vi "5GNR_DPD_AMPM_EVM_ACP_DL.vi"() -> ()   [LabVIEW 2016]
doc: "This example illustrates how to use the RFmx SpecAn and LTE personalities together with the RFSG drivers to perform ACP and EVM measurements with or without digital predistortion (DPD) of the waveform input to the DUT. \n\nDPD is a technique to optimize the operating point of power amplifiers and other non-linear RFIC devices. Power amplifiers are much more efficient if they operate near compression. However, compressing signal amplitudes can significantly deteriorate the amplified signal's quality both, in-band (e.g., EVM increases due to non-linear distortion of the signal's I/Q constellation) and out-of-band (e.g., ACP or SEM test fails due to spectral regrowth). With DPD, the original waveform is first pre-distorted in a way that matches the non-linear effects of the RFIC device before being fed through the device. The resulting output is a much cleaner amplified and/or filtered version of the original waveform. \n\nDifferent DPD models can be used to trade off performance with computational ease, with the Lookup-Table (LUT) model the simplest and the Generalized Memory Polynomial Model (GMP) the most complex. With a LUT, the DPD algorithm achieves gain and phase linearization on average. If you want to correct for memory effects - i.e., an output sample not only depends on the current input but also previous input samples; you will notice that a specific input power value translates into a range of gain and phase values - you would use one of the memory polynomial models. For these models, several parameters such as polynomial order and memory depth are available to fine-tune the model to the DUT behavior."
uses:
  <instrlib>/niRFSG/niRFSG.llb/niRFSG Exported Signal Destinations.ctl
  Source/SG/Typedefs/Instrument Configuration.ctl
  <instrlib>/niRFSG/niRFSG.llb/niRFSG Ref Clock Sources.ctl
  Source/Common/Local Oscillator Sharing Mode.ctl
  Source/Common/SA Common Configuration.ctl
  Source/SA/RFmxNR/Typedefs/NR ACP Configuration.ctl
  Source/SA/RFmxNR/Typedefs/NR ModAcc Configuration.ctl
  Source/SA/RFmxNR/Typedefs/NR ModAcc Component Carrier Results.ctl
  Source/SA/RFmxNR/Typedefs/NR ACP Offset Results.ctl
  Source/SA/RFmxNR/Typedefs/NR ACP Component Carrier Results.ctl
  Source/SA/RFmxSpecAn/Typedefs/SpecAn AMPM Results.ctl
  Source/SA/RFmxSpecAn/Typedefs/SpecAn AMPM Configuration.ctl
  Source/Common/Waveform.ctl
  Source/Methods/RFmxDPD/Typedefs/Common Configuration.ctl
  Source/Methods/RFmxDPD/Typedefs/Memory Polynomial Configuration.ctl
  Source/SA/RFmxInstr/Typedefs/Instrument Configuration.ctl
  Source/Methods/RFmxDPD/Typedefs/Pre DPD Crest Factor Reduction Configuration.ctl
  Source/Methods/RFmxDPD/Typedefs/Pre DPD Crest Factor Reduction Carrier Channel.ctl
  Source/Methods/RFmxDPD/Typedefs/Apply DPD Crest Factor Reduction Configuration.ctl
  Source/Common/SA Auto Level Configuration.ctl
  Source/SA/RFmxNR/Typedefs/NR Standard Configuration.ctl
  <vilib>/RFmx/SpecAn/mx/RFmxSpecAn.llb/RFmxSpecAn AMPM Fetch AM to AM Trace.vi
  <vilib>/RFmx/SpecAn/mx/RFmxSpecAn.llb/RFmxSpecAn AMPM Fetch AM to PM Trace.vi
  <vilib>/RFmx/NR/mx/RFmxNR.llb/RFmxNR ModAcc Fetch PDSCH QPSK Constellation Trace.vi
  <vilib>/RFmx/NR/mx/RFmxNR.llb/RFmxNR ModAcc Fetch RMS EVM per Subcarrier Mean Trace.vi
  <vilib>/RFmx/NR/mx/RFmxNR.llb/RFmxNR ACP Fetch Relative Powers Trace.vi
  <vilib>/RFmx/NR/mx/RFmxNR.llb/RFmxNR ACP Fetch Spectrum.vi
  Source/SG/SG.lvlib
  Source/SA/RFmxNR/RFmxNR.lvlib
  Source/SA/RFmxSpecAn/RFmxSpecAn.lvlib
  Source/Methods/RFmxDPD/RFmxDPD.lvlib
  Source/SA/RFmxInstr/RFmxInstr.lvlib
  Source/Common/Common.lvlib
panel:
  in  "Resource Control":enum32{"RFSG", "5GNR Signal", "RFSA"}(tab)
  in  "Marker Event Output Terminal":T1="PXI_Trig0"
  in  "Reference Waveform File Path":path=path "C:/Users/Public/Documents/National Instruments/RFIC Test Software/Waveforms/NR_FR1_DL_TM1-1_1x100MHz_30kHz-SCS_OS4.tdms"
  in  "RFSG Resource Name":refnum<k15>="RFSG"
  in  "SG Configuration":T2={"SelectedPorts"="", "Reference Clock Source"="PXI_CLK", "Carrier Frequency (Hz)"=3500000000.0, "DUT Average Input Power (dBm)"=-10.0, "External Attenuation (dB)"=0.0, "LO Sharing Mode"=enum."Automatic"}
  in  "Frequency Band":i32=78
  in  "DL TM Duplex Scheme":i32(ring) items=["FDD", "TDD"]
  in  "Downlink TM":i32(ring) items=["TM1.1", "TM1.2", "TM2", "TM2a", "TM3.1", "TM3.1a", "TM3.2", "TM3.3"]
  in  "SA RF (Hz)":dbl=nan format="%.6p"
  in  "RFSA Resource Name":refnum<k15>="RFSA"
  in  "Common Configuration":T5={"Center Frequency (Hz)"=3500000000.0, "Reference Level (dBm)"=0.0, "External Attenuation (dB)"=0.0, "Trigger Enabled"=TRUE, "Digital Trigger Source"="PXI_Trig0", "Trigger Delay (s)"=0.0, "Selected Ports"=""} {"Trigger Delay (s)" format="%.2p"; "External Attenuation (dB)" format="%.2f"; "Reference Level (dBm)" format="%.2f"; "Center Frequency (Hz)" format="%.6p"}
  in  "Instrument Configuration":T6={"LO Sharing Mode"=enum."Automatic", "Frequency Reference Source"="PXI_Clk"}
  in  "Auto Level Configuration":T7={"Enabled"=TRUE, "Measurement Interval (s)"=0.01} {"Measurement Interval (s)" min=1e-06 max=100.0 format="%.2p"}
  in  "Center Frequency / SG IF (Hz)":dbl=3500000000.0 format="%.6p"
  in  "Error Tab Control":enum32{"Page 1", "Page 2"}(tab)
  out "error out":errorcluster
  in  "Display Tab Control":T8(tab)
  out "AM to AM Plot":T9(graph)
  out "AM to PM Plot":T10(graph)
  out "AMPM Measurement Results":T11 {"AM to PM Residual (deg)" format="%.2f"; "AM to AM Residual (dB)" format="%.2f"; "Mean RMS EVM (%)" format="%.2f"; "1 dB Compression Point (dBm)" format="%.2f"; "Mean Linear Gain (dB)" format="%.2f"}
  out "ModAcc Results":cluster{"Component Carrier Results":T12[]}
  out "Constellation Trace":csg[](graph)
  out "EVM Per Subcarrier Trace":cluster{"x0":dbl, "dx":dbl, "y":sgl[]}(graph)
  out "Spectrum":cluster{"x0":dbl, "dx":dbl, "y":sgl[]}[](graph)
  out "ACP Results":T15
  in  "Measurement Settings Tab Control":T16(tab)
  in  "RFmx SpecAn AMPM Configuration":T17={"Measurement Interval (s)"=0.0001, "DUT Average Input Power (dBm)"=-20.0, "Signal Type"=0, "Averaging Enabled"=0, "Averaging Count"=10, "Reference Waveform"={"Name"="Wfm", "Data"=refnum, "Signal Bandwidth (Hz)"=0.0, "PAPR (dB)"=0.0, "Burst Length (s)"=0.0, "Sample Rate"=0.0, "Burst Start Locations"=[], "Burst Stop Locations"=[], "Idle Duration Present?"=FALSE, "Runtime Scaling"=0.0, "Script"=""}} {"Reference Waveform"."Runtime Scaling" format="%#_6p"; "Reference Waveform"."Sample Rate" format="%#_6p"; "Reference Waveform"."Burst Length (s)" format="%#_6p"; "Reference Waveform"."PAPR (dB)" format="%.2f"; "Reference Waveform"."Signal Bandwidth (Hz)" format="%#_6p"; "Averaging Enabled" items=["False", "True"]; "Signal Type" items=["Modulated", "Tones"]; "DUT Average Input Power (dBm)" format="%.2f"; "Measurement Interval (s)" format="%.2p"}
  in  "Common DPD Configuration":T19={"Measurement Interval (s)"=0.0001, "Signal Type"=0, "DUT Average Input Power (dBm)"=-15.0, "Synchronization Method"=1} {"Synchronization Method" items=["Direct"=1, "Alias Protected"=2]; "DUT Average Input Power (dBm)" format="%.2f"; "Signal Type" items=["Modulated", "Tones"]; "Measurement Interval (s)" format="%#.2p"}
  in  "Memory Polynomial Configuration":T20={"Correction Type"=0, "Number of Iterations"=1, " Order"=3, " Depth"=2, "Lead Order"=2, "Lag Order"=2, "Lead Memory Depth"=2, "Lag Memory Depth"=2, "Maximum Lead"=2, "Maximum Lag"=2} {"Order" min=1; "Correction Type" items=["Magnitude and Phase", "Magnitude Only", "Phase Only"]}
  in  "Enable DPD":bool=TRUE
  in  "Pre DPD Crest Factor Reduction":T21={"Enabled"=0, "Method"=0, "Max Iterations"=10, "Target PAPR (dB)"=8.0, "Shaping Factor"=5.0, "Shaping Threshold (dB)"=-5.0, "Window Type"=7, "Window Length"=10, "Filter Enabled"=0, "Carrier Channels"=[{"Offset (Hz)"=0.0, "Bandwidth (Hz)"=20000000.0}]} {"Carrier Channels"."Bandwidth (Hz)" format="%.2p"; "Carrier Channels"."Offset (Hz)" format="%.2p"; "Filter Enabled" items=["False", "True"]; "Window Type" items=["Flat Top"=1, "Hanning"=2, "Hamming"=3, "Gaussian"=4, "Blackman"=5, "Blackman-Harris"=6, "Kaiser-Bessel"=7]; "Method" items=["Clipping", "Peak Windowing", "Sigmoid"]; "Enabled" items=["False", "True"]}
  in  "Apply DPD Crest Factor Reduction":T23={"Enabled"=0, "Method"=0, "Max Iterations"=10, "Target PAPR Type"=0, "Target PAPR (dB)"=8.0, "Window Type"=7, "Window Length"=10, "Shaping Factor"=5.0, "Shaping Threshold (dB)"=-5.0} {"Target PAPR Type" items=["Input PAPR", "Custom"]; "Window Type" items=["Flat Top"=1, "Hanning"=2, "Hamming"=3, "Gaussian"=4, "Blackman"=5, "Blackman-Harris"=6, "Kaiser-Bessel"=7]; "Method" items=["Clipping", "Peak Windowing", "Sigmoid"]; "Enabled" items=["False", "True"]}
  in  "NR ModAcc Configuration":T24={"Measurement Length Unit"=1, "Measurement Offset"=0.0, "Measurement Length"=1.0, "EVM Unit"=0, "Averaging Enabled"=0, "Averaging Count"=10} {"Averaging Enabled" items=["False", "True"]; "EVM Unit" items=["Percentage", "dB"]; "Measurement Length Unit" items=["Slot"=1, "Subframe"=3, "Time"=6]}
  in  "NR ACP Configuration":T25={"Number of UTRA Offsets"=0, "Number of EUTRA Offsets"=0, "Number of NR Offsets"=2, "Number of ENDC Offsets"=0, "Measurement Method"=0, "Noise Compensation Enabled"=0, "Sweep Time Auto"=1, "Sweep Time Interval (s)"=0.001, "Averaging Enabled"=0, "Averaging Count"=10, "Averaging Type"=0} {"Measurement Method" items=["Normal", "Dynamic Range", "Sequential FFT"]; "Noise Compensation Enabled" items=["False", "True"]; "Sweep Time Auto" items=["False", "True"]; "Averaging Type" items=["RMS", "Log", "Scalar", "Max", "Min"]; "Averaging Enabled" items=["False", "True"]}
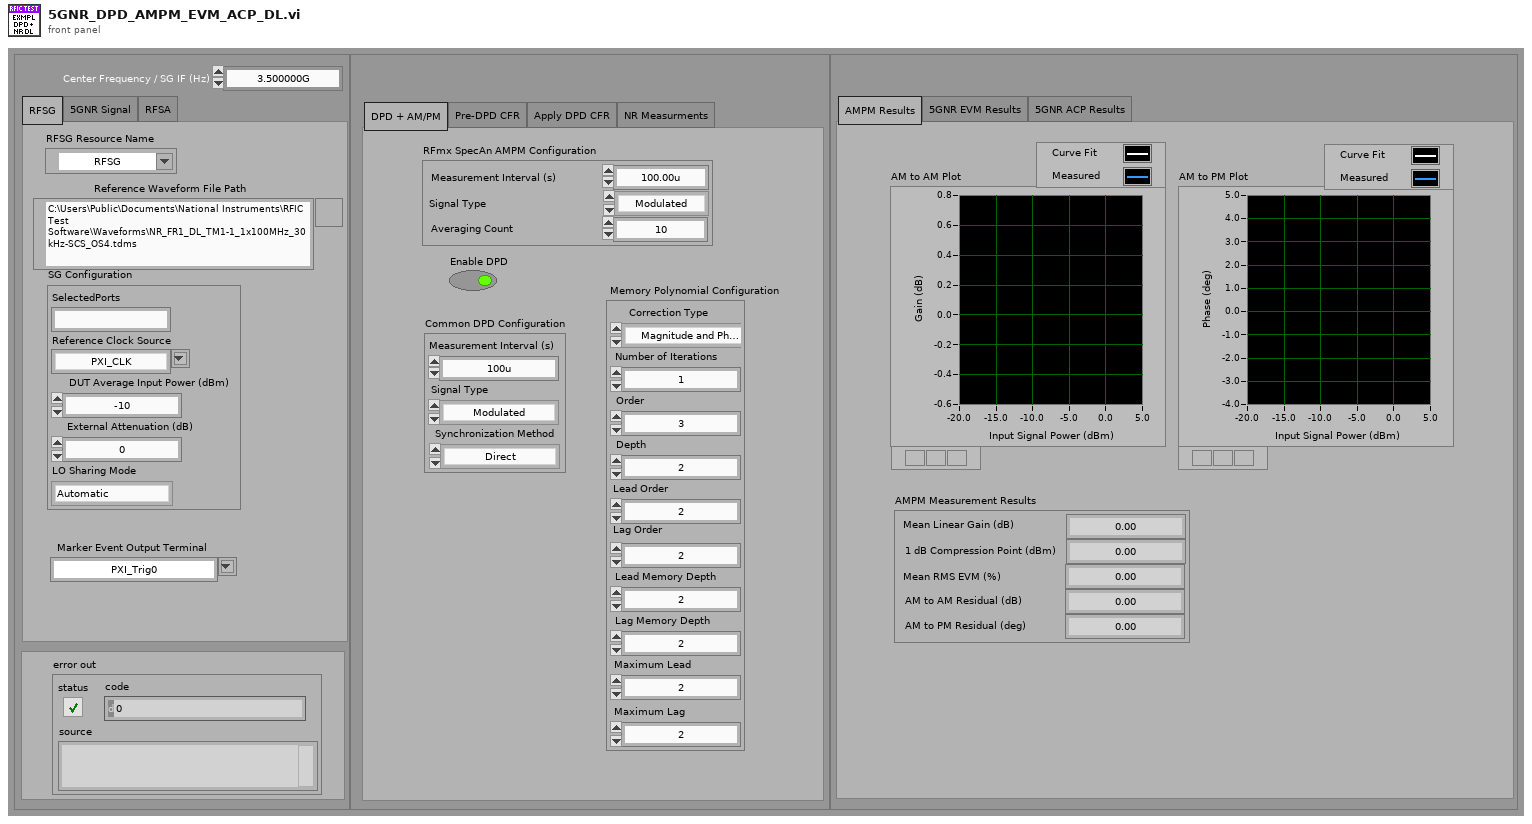
[diagram p1: front panel]
types:
  T1 = typedef "niRFSG Exported Signal Destinations.ctl" = string
  T2 = typedef "SG.lvlib/Instrument Configuration.ctl" = cluster{"SelectedPorts":string, "Reference Clock Source":T3, "Carrier Frequency (Hz)":dbl, "DUT Average Input Power (dBm)":dbl, "External Attenuation (dB)":dbl, "LO Sharing Mode":T4}
  T3 = typedef "niRFSG Ref Clock Sources.ctl" = string
  T4 = typedef "Common.lvlib/Local Oscillator Sharing Mode.ctl" = enum16{"Automatic", "None"}
  T5 = typedef "Common.lvlib/SA Common Configuration.ctl" = cluster{"Center Frequency (Hz)":dbl, "Reference Level (dBm)":dbl, "External Attenuation (dB)":dbl, "Trigger Enabled":bool, "Digital Trigger Source":string, "Trigger Delay (s)":dbl, "Selected Ports":string}
  T6 = typedef "RFmxInstr.lvlib/Instrument Configuration.ctl" = cluster{"LO Sharing Mode":T4, "Frequency Reference Source":string}
  T7 = typedef "Common.lvlib/SA Auto Level Configuration.ctl" = cluster{"Enabled":bool, "Measurement Interval (s)":dbl}
  T8 = enum32{"AMPM Results", "5GNR EVM Results", "5GNR ACP Results"}
  T9 = cluster{"Input Powers (dBm)":sgl[], "Curve Fit AM to AM (dB)":sgl[]}[]
  T10 = cluster{"Input Powers (dBm)":sgl[], "Curve Fit AM to PM (dB)":sgl[]}[]
  T11 = typedef "RFmxSpecAn.lvlib/SpecAn AMPM Results.ctl" = cluster{"Mean Linear Gain (dB)":dbl, "1 dB Compression Point (dBm)":dbl, "Mean RMS EVM (%)":dbl, "AM to AM Residual (dB)":dbl, "AM to PM Residual (deg)":dbl}
  T12 = typedef "RFmxNR.lvlib/NR ModAcc Component Carrier Results.ctl" = cluster{"Peak Composite EVM Subcarrier Index":i32, "Peak Composite EVM Symbol Index":i32, "Mean RMS Composite EVM":dbl, "Max Peak Composite EVM":dbl, "Mean Frequency Error (Hz)":dbl, "Peak Composite EVM Slot Index":i32}
  T13 = typedef "RFmxNR.lvlib/NR ACP Offset Results.ctl" = cluster{"Upper Absolute Power (dBm)":dbl, "Lower Absolute Power (dBm)":dbl, "Lower Relative Power (dB)":dbl, "Upper Relative Power (dB)":dbl, "Frequency (Hz)":dbl, "Integration Bandwidth (Hz)":dbl}
  T14 = typedef "RFmxNR.lvlib/NR ACP Component Carrier Results.ctl" = cluster{"Absolute Power (dBm)":dbl, "Relative Power (dB)":dbl}
  T15 = cluster{"Offset Results":T13[], "Component Carrier Results":T14[]}
  T16 = enum32{"DPD + AM/PM", "Pre-DPD CFR", "Apply DPD CFR", "NR Measurments"}
  T17 = typedef "RFmxSpecAn.lvlib/SpecAn AMPM Configuration.ctl" = cluster{"Measurement Interval (s)":dbl, "DUT Average Input Power (dBm)":dbl, "Signal Type":i32, "Averaging Enabled":i32, "Averaging Count":i32, "Reference Waveform":T18}
  T18 = typedef "Common.lvlib/Waveform.ctl" = cluster{"Name":string, "Data":refnum<data-value>, "Signal Bandwidth (Hz)":dbl, "PAPR (dB)":dbl, "Burst Length (s)":dbl, "Sample Rate":dbl, "Burst Start Locations":i32[], "Burst Stop Locations":i32[], "Idle Duration Present?":bool, "Runtime Scaling":dbl, "Script":string}
  T19 = typedef "RFmxDPD.lvlib/Common Configuration.ctl" = cluster{"Measurement Interval (s)":dbl, "Signal Type":i32, "DUT Average Input Power (dBm)":dbl, "Synchronization Method":i32}
  T20 = typedef "RFmxDPD.lvlib/Memory Polynomial Configuration.ctl" = cluster{"Correction Type":i32, "Number of Iterations":i32, " Order":i32, " Depth":i32, "Lead Order":i32, "Lag Order":i32, "Lead Memory Depth":i32, "Lag Memory Depth":i32, "Maximum Lead":i32, "Maximum Lag":i32}
  T21 = typedef "RFmxDPD.lvlib/Pre DPD Crest Factor Reduction Configuration.ctl" = cluster{"Enabled":i32, "Method":i32, "Max Iterations":i32, "Target PAPR (dB)":dbl, "Shaping Factor":dbl, "Shaping Threshold (dB)":dbl, "Window Type":i32, "Window Length":i32, "Filter Enabled":i32, "Carrier Channels":T22[]}
  T22 = typedef "RFmxDPD.lvlib/Pre DPD Crest Factor Reduction Carrier Channel.ctl" = cluster{"Offset (Hz)":dbl, "Bandwidth (Hz)":dbl}
  T23 = typedef "RFmxDPD.lvlib/Apply DPD Crest Factor Reduction Configuration.ctl" = cluster{"Enabled":i32, "Method":i32, "Max Iterations":i32, "Target PAPR Type":i32, "Target PAPR (dB)":dbl, "Window Type":i32, "Window Length":i32, "Shaping Factor":dbl, "Shaping Threshold (dB)":dbl}
  T24 = typedef "RFmxNR.lvlib/NR ModAcc Configuration.ctl" = cluster{"Measurement Length Unit":i32, "Measurement Offset":dbl, "Measurement Length":dbl, "EVM Unit":i32, "Averaging Enabled":i32, "Averaging Count":i32}
  T25 = typedef "RFmxNR.lvlib/NR ACP Configuration.ctl" = cluster{"Number of UTRA Offsets":i32, "Number of EUTRA Offsets":i32, "Number of NR Offsets":i32, "Number of ENDC Offsets":i32, "Measurement Method":i32, "Noise Compensation Enabled":i32, "Sweep Time Auto":i32, "Sweep Time Interval (s)":dbl, "Averaging Enabled":i32, "Averaging Count":i32, "Averaging Type":i32}
  T26 = enum16{"ModAcc", "SEM", "ACP", "CHP", "OBW", "PVT"}[]
  T27 = enum16{"ACP", "CCDF", "CHP", "FCnt", "Harmonics", "OBW", "SEM", "Spectrum", "Spur", "TXP", "AMPM", "DPD", "IQ", "IM", "NF", "PhaseNoise", "PAVT"}[]
  T28 = typedef "RFmxNR.lvlib/NR Standard Configuration.ctl" = cluster{"Link Direction":i32, "Frequency Range":i32, "Band":i32, "Auto Resource Block Detection Enabled":i32, "Downlink Test Model":i32, "Downlink Test Model Duplex Scheme":i32, "Component Carrier Configurations":cluster{"Bandwidth (Hz)":dbl, "Cell ID":i32, "PUSCH Modulation Type":i32, "Subcarrier Spacing (Hz)":dbl, "PUSCH Resource Block Offset":i32, "PUSCH Number of Resource Blocks":i32, "PUSCH Transform Precoding Enabled":i32, "PUSCH Slot Allocation":string, "PUSCH Symbol Allocation":string, "PUSCH DMRS Configuration Type":i32, "PUSCH Mapping Type":i32, "PUSCH DMRS Type A Position":i32, "PUSCH DMRS Duration":i32, "PUSCH DMRS Additional Positions":i32}[]}
  T29 = cluster{"Reference Powers (dBm)":sgl[], "Curve Fit AM to AM (dB)":sgl[]}
  T30 = cluster{"Reference Powers (dBm)":sgl[], "Measured AM to AM (dB)":sgl[]}
  T31 = cluster{"Reference Powers (dBm)":sgl[], "Curve Fit AM to PM (deg)":sgl[]}
  T32 = cluster{"Reference Powers (dBm)":sgl[], "Measured AM to PM (deg)":sgl[]}
  T33 = cluster{"Reference Powers (dBm)":sgl[], "Measured AM to AM (dB)":sgl[]}[]
  T34 = cluster{"Reference Powers (dBm)":sgl[], "Measured AM to PM (deg)":sgl[]}[]
  T35 = typedef "RFmxNR.lvlib/NR ModAcc Results.ctl" = cluster{"Component Carrier Results":T12[]}
  T36 = typedef "RFmxNR.lvlib/NR ACP Results.ctl" = cluster{"Offset Results":T13[], "Component Carrier Results":T14[]}
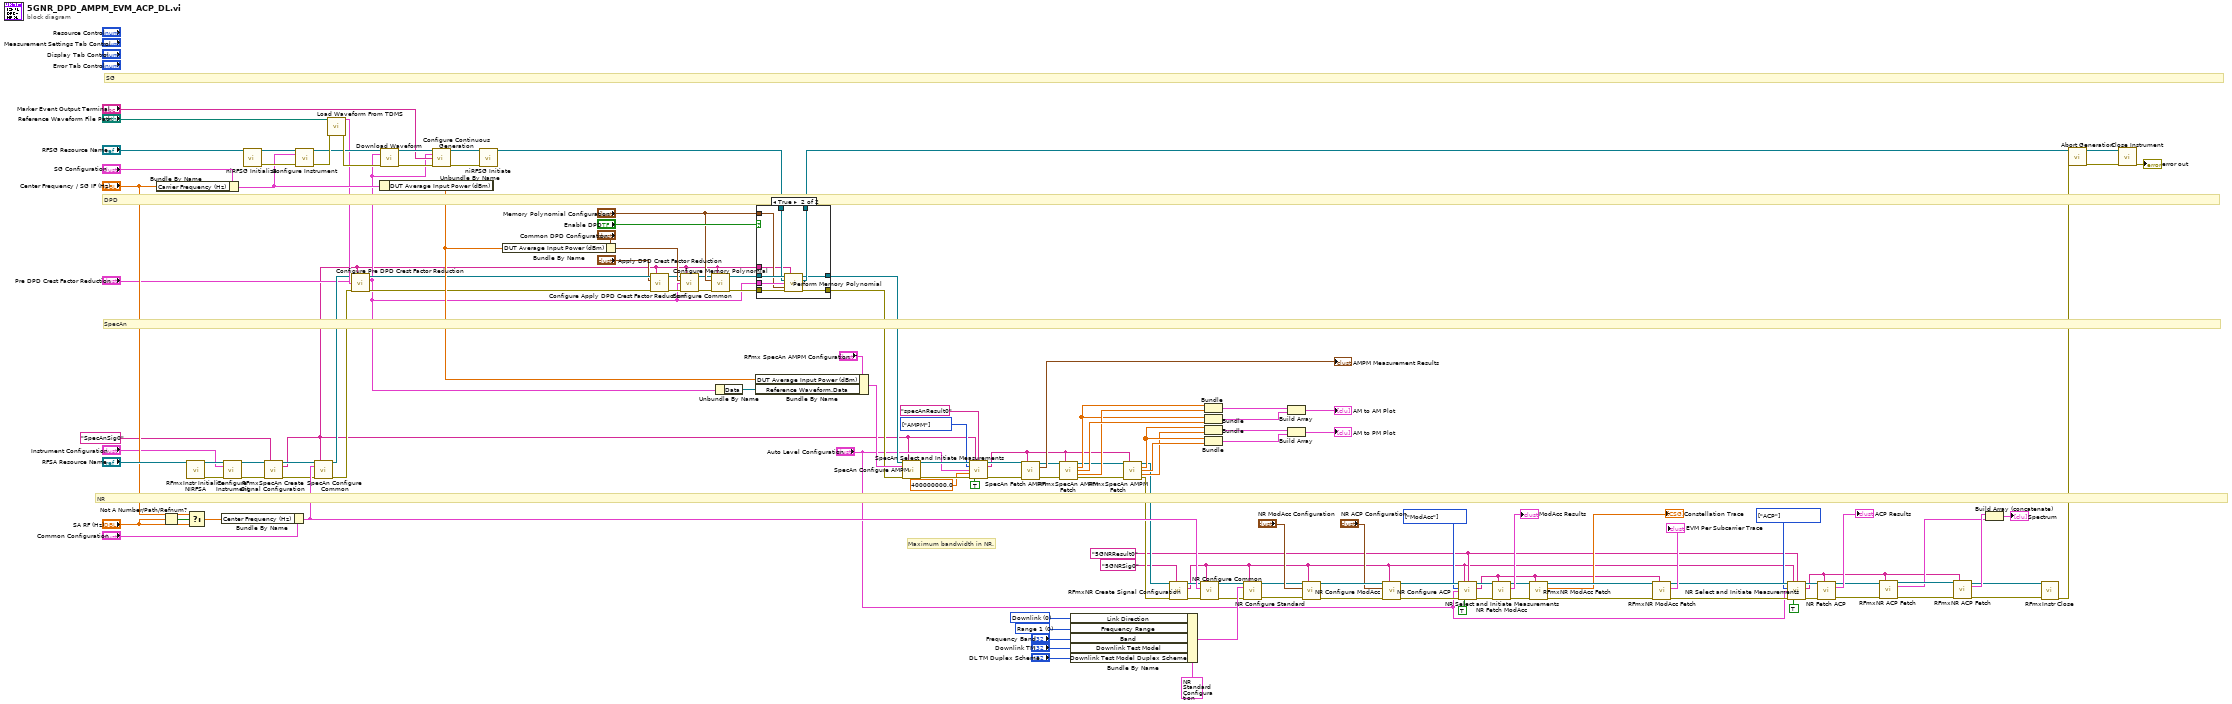
[diagram p0: block diagram]
diagram:
  w8 = "5GNRResult0" ("Signal Name")
  w19 = T26 [enum."ACP"] items=["ModAcc", "SEM", "ACP", "CHP", "OBW", "PVT"] ("Measurements")
  w27 = T26 [enum."ModAcc"] items=["ModAcc", "SEM", "ACP", "CHP", "OBW", "PVT"] ("Measurements")
  w34 = T27 [enum."AMPM"] items=["ACP", "CCDF", "CHP", "FCnt", "Harmonics", "OBW", "SEM", "Spectrum", "Spur", "TXP", "AMPM", "DPD", "IQ", "IM", "NF", "PhaseNoise", "PAVT"] ("Measurements")
  w128 = 0 items=["Range 1", "Range 2"] ("Frequency Range")
  w129 = 0 items=["Downlink", "Uplink"] ("Link Direction")
  # "Maximum bandwidth in NR."
  # "SpecAn"
  # "SG"
  # "DPD"
  # "NR"
  n1 = Bundle By Name(cluster="SG Configuration", "Carrier Frequency (Hz)"="Center Frequency / SG IF (Hz)") -> (w92:T2)
  n2 = Not A Number/Path/Refnum?(number/path/refnum="SA RF (Hz)") -> (NaN/Path/Refnum?=w132:bool)
  n3 = call <vilib>:"RFmxInstr Initialize NIRFSA.vi"("Resource Name"="RFSA Resource Name") -> ("Instrument Handle Out"=w50:refnum<k21>, "error out"=w49:errorcluster)  [unwired: 12 in, 1 out]
  n4 = Select(t="Center Frequency / SG IF (Hz)", s=w132, f="SA RF (Hz)") -> (s? t:f=w117:dbl)
  n5 = Bundle By Name(cluster="Common Configuration", "Center Frequency (Hz)"=w117) -> (w51:T5)
  n6 = call "Configure Instrument.vi"("Instrument Handle In"=w50, "Instrument Configuration"="Instrument Configuration", "error in (no error)"=w49) -> ("Instrument Handle Out"=w17:refnum<k21>, "error out"=w15:errorcluster)  [unwired: 11 in]
  n7 = call <instrlib>:"niRFSG Initialize.vi"("resource name"="RFSG Resource Name") -> ("instrument handle"=w134:refnum<k15>, "error out"=w133:errorcluster)  [unwired: 13 in]
  n8 = call <vilib>:"RFmxSpecAn Create Signal Configuration.vi"("Instrument Handle In"=w17, "Signal Name"="SpecAnSig0", "error in (no error)"=w15) -> ("Instrument Handle Out"=w16:refnum<k21>, "Selector String Out"=w4:string, "error out"=w14:errorcluster)  [unwired: 10 in]
  n9 = call "Configure Instrument.vi"("RFSG Session In"=w134, "SG Configuration"=w92, "error in (no error)"=w133) -> ("RFSG Session Out"=w138:refnum<k15>, "error out"=w140:errorcluster)  [unwired: 11 in]
  n10 = call "SpecAn Configure Common.vi"("RFmx Handle In"=w16, "Selector String"=w4, "Common Configuration"=w51, "error in (no error)"=w14) -> ("RFmx Handle Out"=w42:refnum<k21>, "error out"=w41:errorcluster)  [unwired: 10 in]
  n11 = call "Load Waveform From TDMS.vi"("TDMS File Path"="Reference Waveform File Path", "error in (no error)"=w140) -> ("Waveform"=w47:T18, "error out"=w139:errorcluster)  [unwired: 12 in]
  n12 = call "Configure Pre DPD Crest Factor Reduction.vi"("Instrument Handle In"=w42, "Selector String"=w4, "Pre DPD Crest Factor Reduction Configuration"="Pre DPD Crest Factor Reduction", "Reference Waveform"=w47, "error in (no error)"=w41) -> ("Instrument Handle Out"=w46:refnum<k21>, "Pre DPD CFR Waveform"=w18:T18, "error out"=w43:errorcluster)  [unwired: 8 in]
  n13 = Unbundle By Name(w92) -> ("DUT Average Input Power (dBm)"=w60:dbl)
  n14 = call "Download Waveform.vi"("RFSG handle"=w138, "Waveform In"=w18, "error in (no error)"=w139) -> ("RFSG handle out"=w126:refnum<k15>, "error out"=w124:errorcluster)  [unwired: 11 in]
  n15 = call "Configure Continuous Generation.vi"("RFSG handle"=w126, "Waveform in"=w18, "Waveform Start Trigger Export"="Marker Event Output Terminal", "error in"=w124) -> ("RFSG handle out"=w125:refnum<k15>, "error out"=w123:errorcluster)  [unwired: 9 in, 1 out]
  n16 = call <instrlib>:"niRFSG Initiate.vi"("instrument handle"=w125, "error in"=w123) -> ("instrument handle out"=w62:refnum<k15>)  [unwired: 12 in, 1 out]
  n17 = Bundle By Name(cluster="Common DPD Configuration", "DUT Average Input Power (dBm)"=w60) -> (w56:T19)
  n18 = call "Configure Apply DPD Crest Factor Reduction.vi"("Instrument Handle In"=w46, "Selector String"=w4, "Apply DPD Crest Factor Reduction Configuration"="Apply DPD Crest Factor Reduction", "error in (no error)"=w43) -> ("Instrument Handle Out"=w45:refnum<k21>, "error out"=w44:errorcluster)  [unwired: 10 in]
  n19 = call "Configure Common.vi"("Instrument Handle In"=w45, "Selector String"=w4, "Common Configuration"=w56, "Reference Waveform"=w18, "error in (no error)"=w44) -> ("Instrument Handle Out"=w55:refnum<k21>, "error out"=w59:errorcluster)  [unwired: 9 in]
  n20 = call "Configure Memory Polynomial.vi"("Instrument Handle In"=w55, "Selector String"=w4, "Memory Polynomial Configuration"="Memory Polynomial Configuration", "error in (no error)"=w59) -> ("Instrument Handle Out"=w67:refnum<k21>, "error out"=w66:errorcluster)  [unwired: 10 in]
  n21 = Unbundle By Name(w18) -> ("Data"=w54:refnum<data-value>)
  n22 = Bundle By Name(cluster="RFmx SpecAn AMPM Configuration", "DUT Average Input Power (dBm)"=w60, "Reference Waveform.Data"=w54) -> (w86:T17)
  n23 = case shown="True" "Enable DPD" {
    tunnel: w67 -> [w142 w152]
    tunnel: [w141 w151] -> w52
    tunnel: "Memory Polynomial Configuration" -> [_ w145]
    tunnel: w18 -> [_ w150]
    tunnel: w62 -> [w143 w149]
    tunnel: [w143 w148] -> w61
    tunnel: [w142 w147] -> w53
    tunnel: w66 -> [w141 w146]
    tunnel: w4 -> [_ w144]
    frame False {
    }
    frame True {
      n24 = call "Perform Memory Polynomial.vi"("RFmx Instrument Handle In"=w152, "Selector String"=w144, "RFSG Instrument Handle In"=w149, "Reference Waveform"=w150, "Memory Polynomial Configuration"=w145, "error in (no error)"=w146) -> ("RFmx Instrument Handle Out"=w147:refnum<k21>, "RFSG Instrument Handle Out"=w148:refnum<k15>, "error out"=w151:errorcluster)  [unwired: 6 in, 1 out]
    }
  }
  n25 = call "SpecAn Configure AMPM.vi"("RFmx Handle In"=w53, "Selector String"=w4, "RFmx SpecAn AMPM Configuration"=w86, "error in (no error)"=w52) -> ("RFmx Handle Out"=w38:refnum<k21>, "error out"=w36:errorcluster)  [unwired: 10 in]
  n26 = call "SpecAn Select and Initiate Measurements.vi"("Instrument Handle In"=w38, "Selector String"=w4, "Result Name"="specAnResult0", "Measurements"=w34, "Auto Level Configuration"="Auto Level Configuration", "Auto Level Bandwidth (Hz)"=400000000.0, "error in (no error)"=w36, "Enable All Traces (F)"=TRUE) -> ("Instrument Handle Out"=w37:refnum<k21>, "Selector String Out"=w2:string, "error out"=w35:errorcluster)  [unwired: 5 in]
  n27 = call "SpecAn Fetch AMPM.vi"("RFmx Handle In"=w37, "Selector String"=w2, "error in (no error)"=w35) -> ("RFmx Handle Out"=w69:refnum<k21>, "AMPM Results"=→"AMPM Measurement Results":T11, "error out"=w72:errorcluster)  [unwired: 10 in]
  n28 = call-poly <vilib>:"RFmxSpecAn AMPM Fetch.vi"("Instrument Handle In"=w69, "Selector String"=w2, "error in (no error)"=w72) -> ("Instrument Handle Out"=w78:refnum<k21>, "Reference Powers (dBm)"=w82:sgl[], "Measured AM to AM (dB)"=w84:sgl[], "Curve Fit AM to AM (dB)"=w83:sgl[], "error out"=w77:errorcluster)  [unwired: 8 in]
  n29 = Bundle By Name(cluster=T28 {"Link Direction"=1, "Frequency Range"=0, "Band"=78, "Auto Resource Block Detection Enabled"=1, "Downlink Test Model"=0, "Downlink Test Model Duplex Scheme"=0, "Component Carrier Configurations"=[{"Bandwidth (Hz)"=100000000.0, "Cell ID"=0, "PUSCH Modulation Type"=1, "Subcarrier Spacing (Hz)"=30000.0, "PUSCH Resource Block Offset"=0, "PUSCH Number of Resource Blocks"=-1, "PUSCH Transform Precoding Enabled"=0, "PUSCH Slot Allocation"="0-Last", "PUSCH Symbol Allocation"="0-Last", "PUSCH DMRS Configuration Type"=0, "PUSCH Mapping Type"=0, "PUSCH DMRS Type A Position"=2, "PUSCH DMRS Duration"=1, "PUSCH DMRS Additional Positions"=0}]} ("NR Signal Configuration"), "Link Direction"=w129, "Frequency Range"=w128, "Band"="Frequency Band", "Downlink Test Model"="Downlink TM", "Downlink Test Model Duplex Scheme"="DL TM Duplex Scheme") -> (w130:T28)
  n30 = call-poly <vilib>:"RFmxSpecAn AMPM Fetch.vi"("Instrument Handle In"=w78, "Selector String"=w2, "error in (no error)"=w77) -> ("Instrument Handle Out"=w12:refnum<k21>, "Reference Powers (dBm)"=w81:sgl[], "Measured AM to PM (deg)"=w80:sgl[], "Curve Fit AM to PM (deg)"=w79:sgl[], "error out"=w9:errorcluster)  [unwired: 8 in]
  n31 = call <vilib>:"RFmxNR Create Signal Configuration.vi"("Instrument Handle In"=w12, "Signal Name"="5GNRSig0", "error in (no error)"=w9) -> ("Instrument Handle Out"=w11:refnum<k21>, "Selector String Out"=w1:string, "error out"=w10:errorcluster)  [unwired: 10 in]
  n32 = call "NR Configure Common.vi"("RFmx Handle In"=w11, "Selector String"=w1, "Common Configuration"=w51, "error in (no error)"=w10) -> ("RFmx Handle Out"=w58:refnum<k21>, "error out"=w57:errorcluster)  [unwired: 10 in]
  n33 = Bundle("Reference Powers (dBm)"=w82, "Curve Fit AM to AM (dB)"=w83) -> (w76:T29)  [unwired: 1 in]
  n34 = Bundle("Reference Powers (dBm)"=w82, "Measured AM to AM (dB)"=w84) -> (w75:T30)  [unwired: 1 in]
  n35 = Bundle("Reference Powers (dBm)"=w81, "Curve Fit AM to PM (deg)"=w79) -> (w73:T31)  [unwired: 1 in]
  n36 = Bundle("Reference Powers (dBm)"=w81, "Measured AM to PM (deg)"=w80) -> (w74:T32)  [unwired: 1 in]
  n37 = call "NR Configure Standard.vi"("RFmx Handle In"=w58, "Selector String"=w1, "NR Standard Configuration"=w130, "error in (no error)"=w57) -> ("RFmx Handle Out"=w90:refnum<k21>, "error out"=w91:errorcluster)  [unwired: 10 in]
  n38 = Build Array(w76, w75) -> (→"AM to AM Plot":T33)
  n39 = Build Array(w73, w74) -> (→"AM to PM Plot":T34)
  n40 = call "NR Configure ModAcc.vi"("RFmx Handle In"=w90, "Selector String"=w1, "NR ModAcc Configuration"="NR ModAcc Configuration", "error in (no error)"=w91) -> ("RFmx Handle Out"=w122:refnum<k21>, "error out"=w121:errorcluster)  [unwired: 10 in]
  n41 = call "NR Configure ACP.vi"("RFmx Handle In"=w122, "Selector String"=w1, "NR ACP Configuration"="NR ACP Configuration", "error in (no error)"=w121) -> ("RFmx Handle Out"=w31:refnum<k21>, "error out"=w30:errorcluster)  [unwired: 10 in]
  n42 = call "NR Select and Initiate Measurements.vi"("Instrument Handle In"=w31, "Selector String"=w1, "Result Name"=w8, "Measurements"=w27, "Auto Level Configuration"="Auto Level Configuration", "error in (no error)"=w30, "Enable All Traces (F)"=TRUE) -> ("Instrument Handle Out"=w28:refnum<k21>, "Selector String Out"=w7:string, "error out"=w29:errorcluster)  [unwired: 6 in]
  n43 = call "NR Fetch ModAcc.vi"("RFmx Handle In"=w28, "Selector String"=w7, "error in (no error)"=w29) -> ("RFmx Handle Out"=w95:refnum<k21>, "ModAcc Results"=→"ModAcc Results":T35, "error out"=w94:errorcluster)  [unwired: 10 in]
  n44 = call-poly <vilib>:"RFmxNR ModAcc Fetch.vi"("Instrument Handle In"=w95, "Selector String"=w7, "error in (no error)"=w94) -> ("Instrument Handle Out"=w109:refnum<k21>, "QPSK Constellation"=→"Constellation Trace":csg[], "error out"=w110:errorcluster)  [unwired: 10 in]
  n45 = call-poly <vilib>:"RFmxNR ModAcc Fetch.vi"("Instrument Handle In"=w109, "Selector String"=w7, "error in (no error)"=w110) -> ("Instrument Handle Out"=w24:refnum<k21>, "RMS EVM per Subcarrier Mean (% or dB)"=→"EVM Per Subcarrier Trace":cluster{"x0":dbl, "dx":dbl, "y":sgl[]}, "error out"=w23:errorcluster)  [unwired: 10 in]
  n46 = call "NR Select and Initiate Measurements.vi"("Instrument Handle In"=w24, "Selector String"=w1, "Result Name"=w8, "Measurements"=w19, "Auto Level Configuration"="Auto Level Configuration", "error in (no error)"=w23, "Enable All Traces (F)"=TRUE) -> ("Instrument Handle Out"=w25:refnum<k21>, "Selector String Out"=w5:string, "error out"=w22:errorcluster)  [unwired: 6 in]
  n47 = call "NR Fetch ACP.vi"("RFmx Handle In"=w25, "Selector String"=w5, "error in (no error)"=w22) -> ("RFmx Handle Out"=w100:refnum<k21>, "ACP Results"=→"ACP Results":T36, "error out"=w99:errorcluster)  [unwired: 10 in]
  n48 = call-poly <vilib>:"RFmxNR ACP Fetch.vi"("Instrument Handle In"=w100, "Selector String"=w5, "error in (no error)"=w99) -> ("Instrument Handle Out"=w105:refnum<k21>, "Relative Powers (dB)"=w102:cluster{"x0":dbl, "dx":dbl, "y":sgl[]}[], "error out"=w104:errorcluster)  [unwired: 10 in]
  n49 = call-poly <vilib>:"RFmxNR ACP Fetch.vi"("Instrument Handle In"=w105, "Selector String"=w5, "error in (no error)"=w104) -> ("Instrument Handle Out"=w98:refnum<k21>, "Spectrum (dBm)"=w103:cluster{"x0":dbl, "dx":dbl, "y":sgl[]}, "error out"=w97:errorcluster)  [unwired: 10 in]
  n50 = Build Array (concatenate)(w103, w102) -> (→"Spectrum":cluster{"x0":dbl, "dx":dbl, "y":sgl[]}[])
  n51 = call <vilib>:"RFmxInstr Close.vi"("Instrument Handle In"=w98, "error in (no error)"=w97) -> ("error out"=w96:errorcluster)  [unwired: 13 in]
  n52 = call "Abort Generation.vi"("RFSG handle"=w61, "error in (no error)"=w96) -> ("RFSG handle out"=w137:refnum<k15>, "error out"=w136:errorcluster)  [unwired: 12 in]
  n53 = call "Close Instrument.vi"("RFSG Handle"=w137, "error in (no error)"=w136) -> ("error out"=→"error out":errorcluster)  [unwired: 13 in]
